vi "TDK-Lambda GEN LAN Series - Getting Started.vi"() -> ()   [LabVIEW 2025]
doc: "Demonstrates the basic operation of the Lambda Genesys series DC Power Supply using the Ethernet (LAN) connection. \n\nCommands sent to reflect the control settings:\n1. Sets the output voltage and current limits.\n2. Turns the output on.\n3. Waits for the output to settle.\n4. Measures the output voltage and current."
uses:
  <userlib>/TDK-Lambda GEN LAN Series/TDK-Lambda GEN LAN Series.lvlib
panel:
  in  "Slave Address":i32=-1 min=-1 max=30 step=1
  in  "Reset (T)":bool=TRUE
  in  "Output On (T)":bool=TRUE
  out "Output Current":dbl format="%.4f"
  in  "Current Limit":dbl format="%.4f"
  out "Output Voltage":dbl format="%.4f"
  in  "Voltage Limit":dbl format="%.4f"
  in  "Settle (mS)":u32=1000
  in  "VISA":refnum<visa-resource-name>
  # "TDK-Lambda Genesys \n LAN\n  DC Power Supplies"
  # "Getting Started:\nConfigure and Read Once"
  # "Right-Click any control\nto see it's Description"
  # "WAIT"
  # "MEASURE"
  # "CONFIGURE"
  # "(c) 2019 TDK-Lambda.  ALL RIGHTS RESERVED."
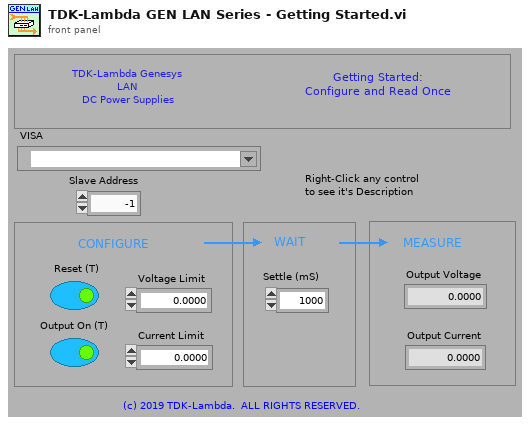
[diagram p1: front panel]
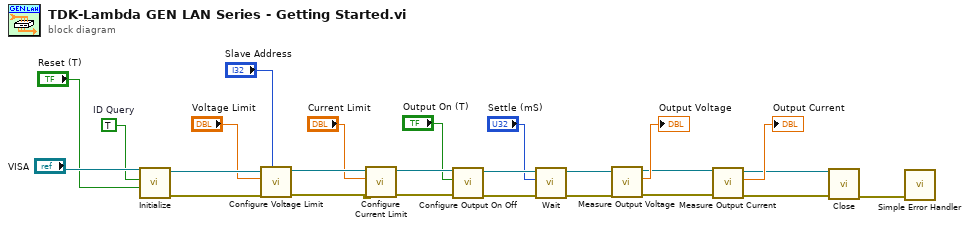
[diagram p0: block diagram]
diagram:
  w24 = TRUE  # ID Query
  n1 = call <userlib>:"Initialize.vi"("Reset (T)"="Reset (T)", "ID Query (T)"=w24, "VISA name"="VISA") -> ("error out"=w22:errorcluster, "VISA out"=w23:refnum<visa-resource-name>)  [unwired: 7 in]
  n2 = call <userlib>:"Configure Voltage Limit.vi"("Slave Address"="Slave Address", "error"=w22, "Voltage Limit"="Voltage Limit", "VISA"=w23) -> ("error out"=w19:errorcluster, "VISA out"=w20:refnum<visa-resource-name>)  [unwired: 6 in]
  n3 = call <userlib>:"Configure Current Limit.vi"("error"=w19, "Current Limit"="Current Limit", "VISA"=w20) -> ("error out"=w16:errorcluster, "VISA out"=w17:refnum<visa-resource-name>)  [unwired: 7 in]
  n4 = call <userlib>:"Configure Output On Off.vi"("error"=w16, "Output ON"="Output On (T)", "VISA"=w17) -> ("error out"=w14:errorcluster, "VISA out"=w15:refnum<visa-resource-name>)  [unwired: 7 in]
  n5 = call <userlib>:"Wait.vi"("error"=w14, "Delay (20 mS)"="Settle (mS)", "VISA"=w15) -> ("error out"=w11:errorcluster, "VISA out"=w12:refnum<visa-resource-name>)  [unwired: 7 in]
  n6 = call <userlib>:"Measure Output Voltage.vi"("error"=w11, "VISA"=w12) -> ("error out"=w9:errorcluster, "Output Voltage"=→"Output Voltage":dbl, "VISA out"=w5:refnum<visa-resource-name>)  [unwired: 7 in]
  n7 = call <userlib>:"Measure Output Current.vi"("error"=w9, "VISA"=w5) -> ("error out"=w3:errorcluster, "Output Current"=→"Output Current":dbl, "VISA out"=w4:refnum<visa-resource-name>)  [unwired: 7 in]
  n8 = call <userlib>:"Close.vi"("error"=w3, "VISA name"=w4) -> ("error out"=w2:errorcluster)  [unwired: 9 in]
  n9 = call <vilib>:"Simple Error Handler.vi"("error in (no error)"=w2) -> ()  [unwired: 4 in, 5 out]
